vi "getFolderID.vi"() -> (0 "error out":errorcluster)   [LabVIEW 2017]
uses:
  Globals/measurementGlobal.vi
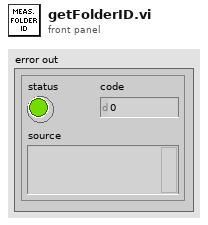
[diagram p1: front panel]
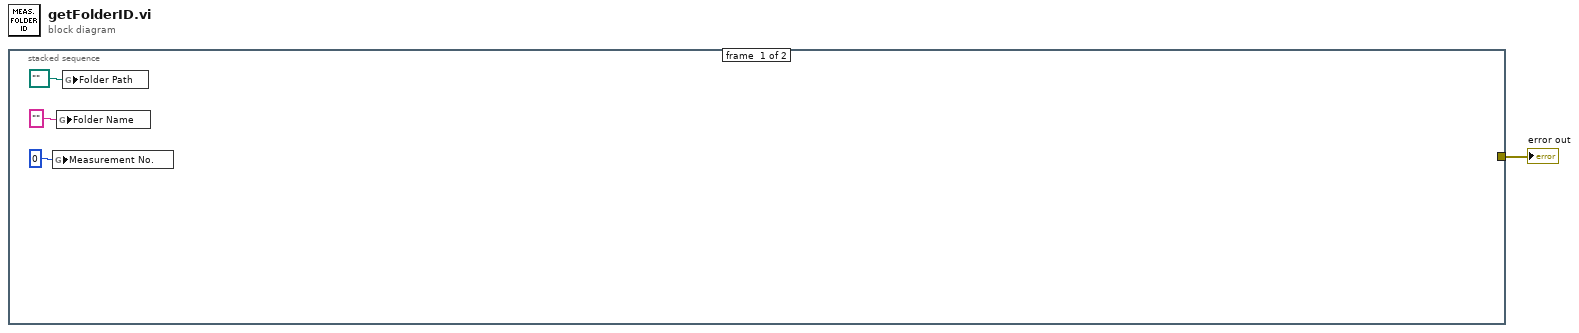
[diagram p0: block diagram]
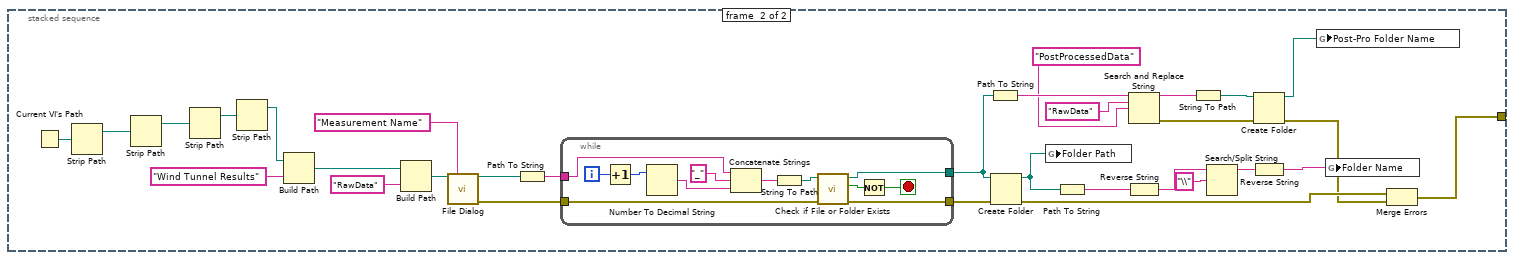
[diagram p2: hidden frame]
diagram:
  n1 = stacked-sequence {
    tunnel: [_ w6] -> w1
    frame #0 {
      n2 = global write "measurementGlobal.vi" "Measurement No."(0 ("Measurement No.")) -> ()
      n3 = global write "measurementGlobal.vi" "Folder Name"("" ("Folder Name")) -> ()
      n4 = global write "measurementGlobal.vi" "Folder Path"(path "" ("Folder Path")) -> ()
    }
    frame #1 {
      n5 = Current VI's Path() -> (path=w35:path)
      n6 = Strip Path(path=w35) -> (stripped path=w34:path)  [unwired: 1 out]
      n7 = Strip Path(path=w34) -> (stripped path=w33:path)  [unwired: 1 out]
      n8 = Strip Path(path=w33) -> (stripped path=w28:path)  [unwired: 1 out]
      n9 = Strip Path(path=w28) -> (stripped path=w27:path)  [unwired: 1 out]
      n10 = Build Path(base path=w27, name or relative path="Wind Tunnel Results") -> (appended path=w16:path)
      n11 = Build Path(base path=w16, name or relative path="RawData") -> (appended path=w30:path)
      n12 = call "File Dialog"("start path"=w30, "prompt"="Measurement Name" ("default name")) -> ("selected path"=w20:path, "error out"=w18:errorcluster)  [unwired: 10 in, 2 out]
      n13 = Path To String(path=w20) -> (string=w19:string)
      n14 = while {
        tunnel: w19 -> [w45]
        tunnel: [w40] -> w15
        tunnel: w18 -> [w37]
        tunnel: [w36] -> w17
        i -> [w47]
        stop <- w39 stop-if-true
        n15 = Increment(x=w47) -> (x+1=w46:i32)
        n16 = Number To Decimal String(number=w46) -> (decimal integer string=w43:string)  [unwired: 1 in]
        n17 = Concatenate Strings(w45, "_" ("string"), w43) -> (w42:string)
        n18 = String To Path(string=w42) -> (path=w41:path)
        n19 = call <vilib>:"Check if File or Folder Exists.vi"("error in (no error)"=w37, "path"=w41) -> ("error out"=w36:errorcluster, "file or folder exists?"=w38:bool, "dup path"=w40:path)  [unwired: 7 in]
        n20 = Not(x=w38) -> (.not. x?=w39:bool)
      }
      n21 = Path To String(path=w15) -> (string=w14:string)
      n22 = Create Folder(path (use dialog)=w15, error in=w17) -> (created path=w22:path, error out=w8:errorcluster)  [unwired: 1 in, 1 out]
      n23 = global write "measurementGlobal.vi" "Folder Path"(w22) -> ()
      n24 = Path To String(path=w22) -> (string=w26:string)
      n25 = Search and Replace String(input string=w14, search string="RawData", replace string="PostProcessedData" ("replace string (\"\")")) -> (result string=w10:string, error out=w11:errorcluster)  [unwired: 5 in, 2 out]
      n26 = Reverse String(1:w26) -> (0:w25:string)
      n27 = String To Path(string=w10) -> (path=w9:path)
      n28 = Search/Split String(string=w25, search string/char (-)="\\") -> (substring before match=w23:string)  [unwired: 1 in, 2 out]
      n29 = Create Folder(path (use dialog)=w9, error in=w11) -> (created path=w5:path, error out=w7:errorcluster)  [unwired: 1 in, 1 out]
      n30 = Reverse String(1:w23) -> (0:w21:string)
      n31 = global write "measurementGlobal.vi" "Post-Pro Folder Name"(w5) -> ()
      n32 = global write "measurementGlobal.vi" "Folder Name"(w21) -> ()
      n33 = Merge Errors(w8, w7) -> (w6:errorcluster)
    }
  }
  "error out" <- w1
